vi "create Behaviour.vi"(8 "error in (no error)":errorcluster caption="Fehler (Eingang, kein Fehler)", 11 "HF-Felder Eingang":refnum<class "HF-Felder.lvclass"> caption="DNL_LabVIEW Object in") -> (0 "error out":errorcluster caption="Fehler (Ausgang)", 1 "regex":string[](array[string]), 2 "response":bool[](array[boolean]), 3 "HF-Felder Ausgang":refnum<class "HF-Felder.lvclass"> caption="DNL_LabVIEW Object out")   [LabVIEW 2013, in "HF-Felder.lvclass"]
uses:
  HF-Felder.lvclass
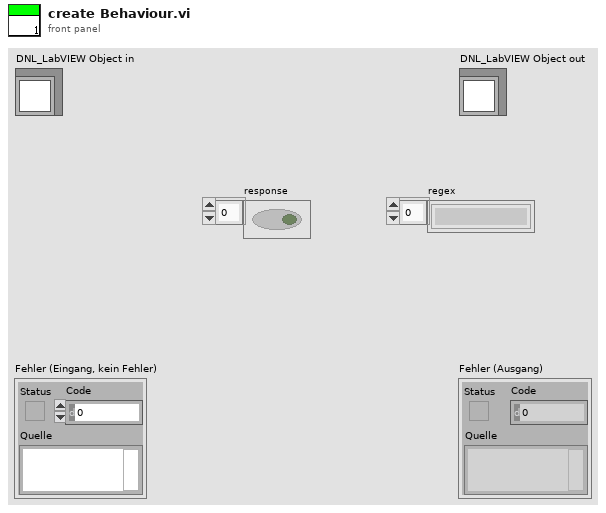
[diagram p1: front panel]
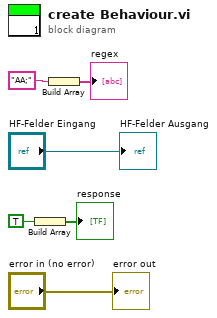
[diagram p0: block diagram]
diagram:
  n1 = Build Array(TRUE) -> (→"response":bool[])
  n2 = Build Array("AA;") -> (→"regex":string[])
  "error out" <- "error in (no error)"
  "HF-Felder Ausgang" <- "HF-Felder Eingang"
